vi "流动字幕.vi"(1 "text":string caption="文本", 5 "模式选择":bool, 6 "日期格式(0)":enum16{"short", "long", "abbreviated"}(ring), 7 "纬度限制1":dbl, 8 "停止":bool, 9 "需要秒？(F)":bool, 10 "等待":u32, 11 "纬度限制 2":dbl) -> (0 "实际纬度1":dbl, 2 "1-bit pixmap   3":bool[][](array[boolean]) caption="固定字幕", 3 "实际纬度 2":dbl, 4 "1-bit pixmap   2":bool[][](array[boolean]) caption="滚动字幕")   [LabVIEW 2014]
panel:
  # "功能菜单"
  # "1.选择默认纬度为100，根据文本长度进行修订。\n2.等待默认为50\n3.模式开关向左，滚动字幕有左向右。"
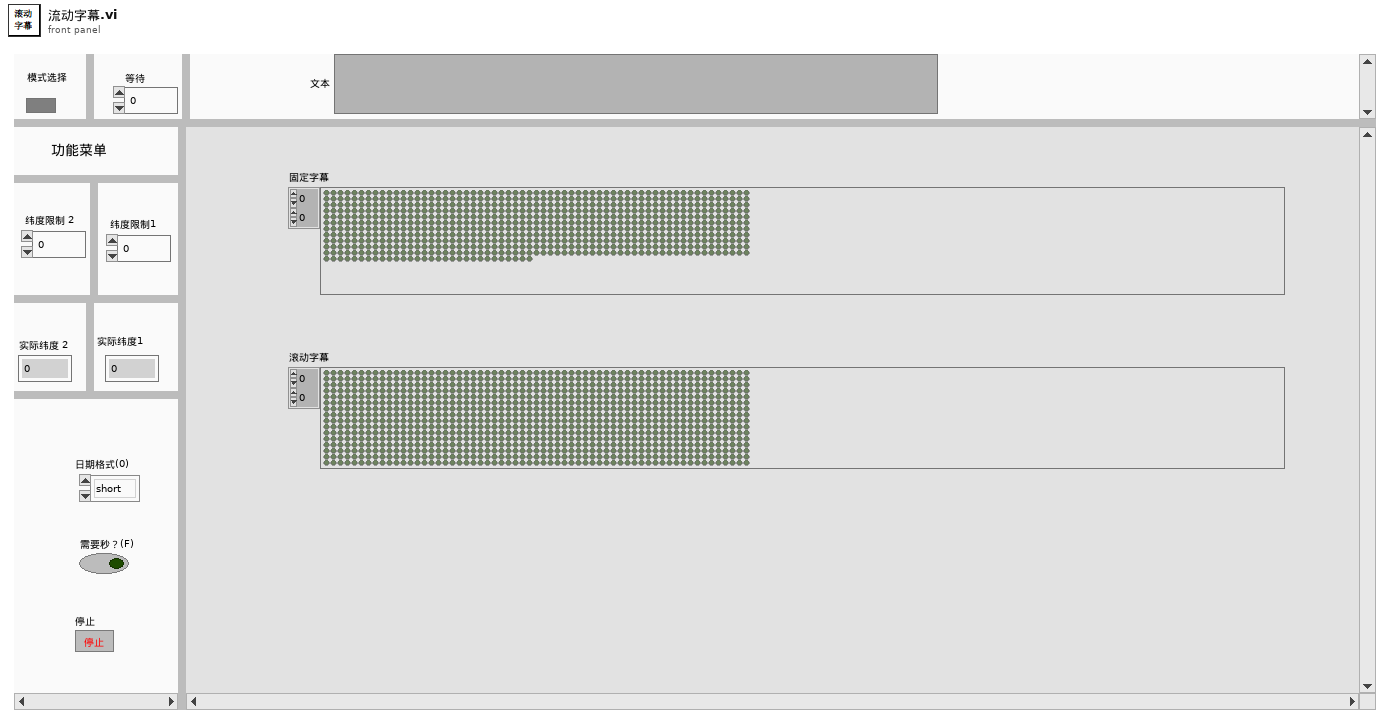
[diagram p1: front panel]
types:
  T1 = cluster{"left":i16, "top":i16, "right":i16, "bottom":i16}
  T2 = typedef "imagedata.ctl" = cluster{"image type":i32, "image depth":i32, "image":u8[], "mask":u8[], "colors":u32[], "Rectangle":cluster{"left":i16, "top":i16, "right":i16, "bottom":i16}}
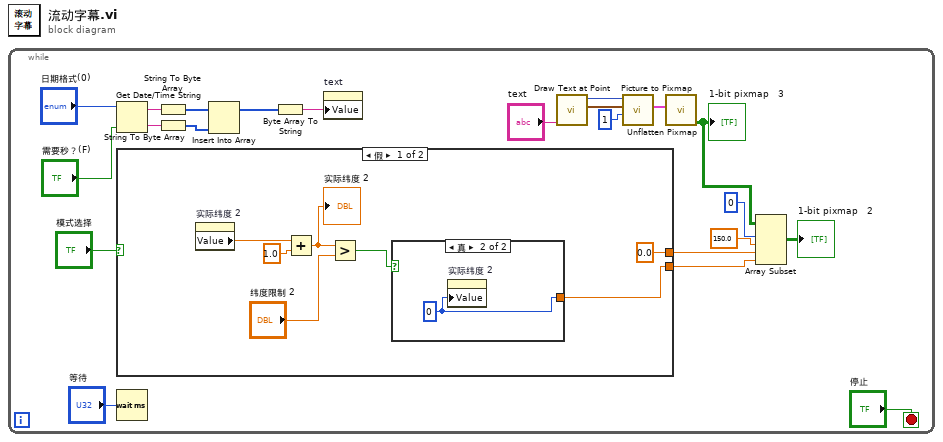
[diagram p0: block diagram]
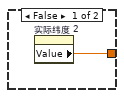
[diagram p2: hidden frame]
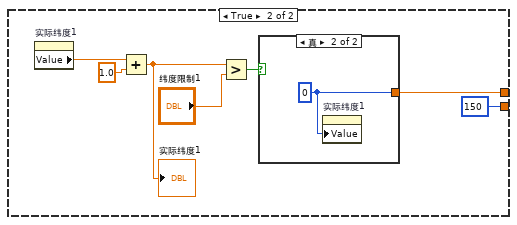
[diagram p3: hidden frame]
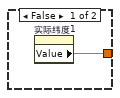
[diagram p4: hidden frame]
diagram:
  n1 = while {
    stop <- "停止" stop-if-true
    n2 = Get Date/Time String(date format (0)="日期格式(0)", want seconds? (F)="需要秒？(F)") -> (date string=w15:string, time string=w17:string)  [unwired: 1 in]
    n3 = case shown="假" "模式选择" {
      tunnel: [0.0 ("y") w33] -> w11
      tunnel: [w23 150 ("长度")] -> w12
      frame False {
        n4 = property on="实际纬度 2" class="DigNum (严格)"() -> ("Value"=w25:dbl)  [unwired: 2 in, 2 out]
        n5 = Add(x=w25, y=1.0) -> (x+y=w28:dbl)
        "实际纬度 2" <- w28
        n6 = Greater?(x=w28, y="纬度限制 2") -> (0:w26:bool)
        n7 = case shown="真" w26 {
          tunnel: [w30 w31] -> w23
          frame False {
            n8 = property on="实际纬度 2" class="DigNum (严格)"() -> ("Value"=w30:dbl)  [unwired: 2 in, 2 out]
          }
          frame True {
            w31 = 0
            n9 = property on="实际纬度 2" class="DigNum (严格)"("Value"=w31) -> ()  [unwired: 2 in, 2 out]
          }
        }
      }
      frame True {
        n10 = property on="实际纬度1" class="DigNum (严格)"() -> ("Value"=w38:dbl)  [unwired: 2 in, 2 out]
        n11 = Add(x=w38, y=1.0) -> (x+y=w35:dbl)
        "实际纬度1" <- w35
        n12 = Greater?(x=w35, y="纬度限制1") -> (0:w37:bool)
        n13 = case shown="真" w37 {
          tunnel: [w39 w40] -> w33
          frame False {
            n14 = property on="实际纬度1" class="DigNum (严格)"() -> ("Value"=w39:dbl)  [unwired: 2 in, 2 out]
          }
          frame True {
            w40 = 0
            n15 = property on="实际纬度1" class="DigNum (严格)"("Value"=w40) -> ()  [unwired: 2 in, 2 out]
          }
        }
      }
    }
    n16 = Wait (ms)(milliseconds to wait="等待") -> ()  [unwired: 1 out]
    n17 = String To Byte Array(string=w15) -> (unsigned byte array=w16:u8[])
    n18 = String To Byte Array(string=w17) -> (unsigned byte array=w18:u8[])
    n19 = Insert Into Array(array=w16, new element=w18) -> (w20:u8[])  [unwired: 1 in]
    n20 = Byte Array To String(unsigned byte array=w20) -> (string=w19:string)
    n21 = property on="text" class="Str"("Value"=w19) -> ()  [unwired: 2 in, 2 out]
    n22 = call <vilib>:"Draw Text at Point.vi"("text"="text") -> ("text rect"=w4:T1, "new picture"=w3:picture)  [unwired: 9 in]
    n23 = call <vilib>:"Picture to Pixmap.vi"("depth"=1, "rect"=w4, "picture"=w3) -> ("image data"=w5:T2)  [unwired: 7 in, 1 out]
    n24 = call <vilib>:"Unflatten Pixmap.vi"("image data"=w5) -> ("1-bit pixmap"=w14:bool[][])  [unwired: 4 in, 6 out]
    "1-bit pixmap   3" <- w14
    n25 = Array Subset(array=w14, index (row)=0 ("索引"), length (row)=150.0 ("y"), index (col)=w11, length (col)=w12) -> (→"1-bit pixmap   2":bool[][])
  }
